vi "mini_test_app_serial_gpib.vi"() -> ()   [LabVIEW 2015]
doc: "Mini test app"
uses:
  Type Definitions/Highway_GB_Data.ctl
  Type Definitions/Highway_HP_Data.ctl
panel:
  out "HP ID":string="\r\n" caption="Hi-Pot Instrument ID"
  out "GB ID":string="\r\n" caption="GB Instrument ID"
  out "I/F type":string caption="Interface type"
  out "Results GB":string
  out "Status GB":string
  in  "Stop GB":bool
  in  "Start GB":bool
  in  "Stop Hi-Pot":bool
  out "Results HP":string
  in  "Exit Button":bool
  in  "Start Hi-Pot":bool
  out "Status HP":string
  # "Warning. This app is a proof of concept and has no other purpose, \nit is not intended for production. Likewise, it has no error handling. \nUse at your own risk."
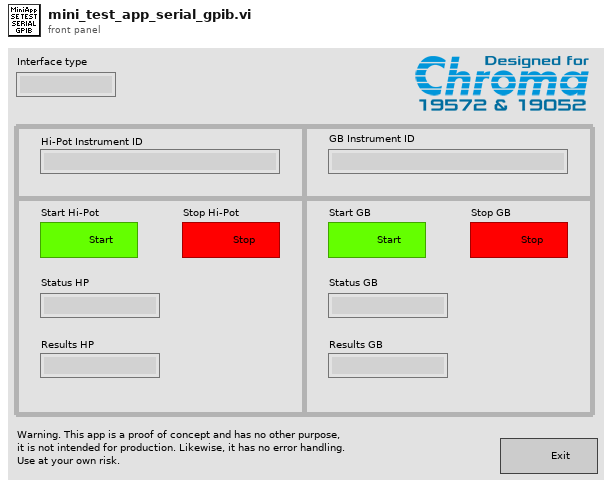
[diagram p1: front panel]
types:
  T1 = typedef "Highway_HP_Data.ctl" = cluster{"Status HP":string, "Results HP":string}
  T2 = typedef "Highway_GB_Data.ctl" = cluster{"Status GB":string, "Results GB":string}
  T3 = cluster{"VISA1 Inst ID":string, "VISA2 Inst ID":string, "I/F type":string}
  T4 = cluster{"Rsrc name for 19572":refnum<visa-resource-name>, "Rsrc name for 19052":refnum<visa-resource-name>}
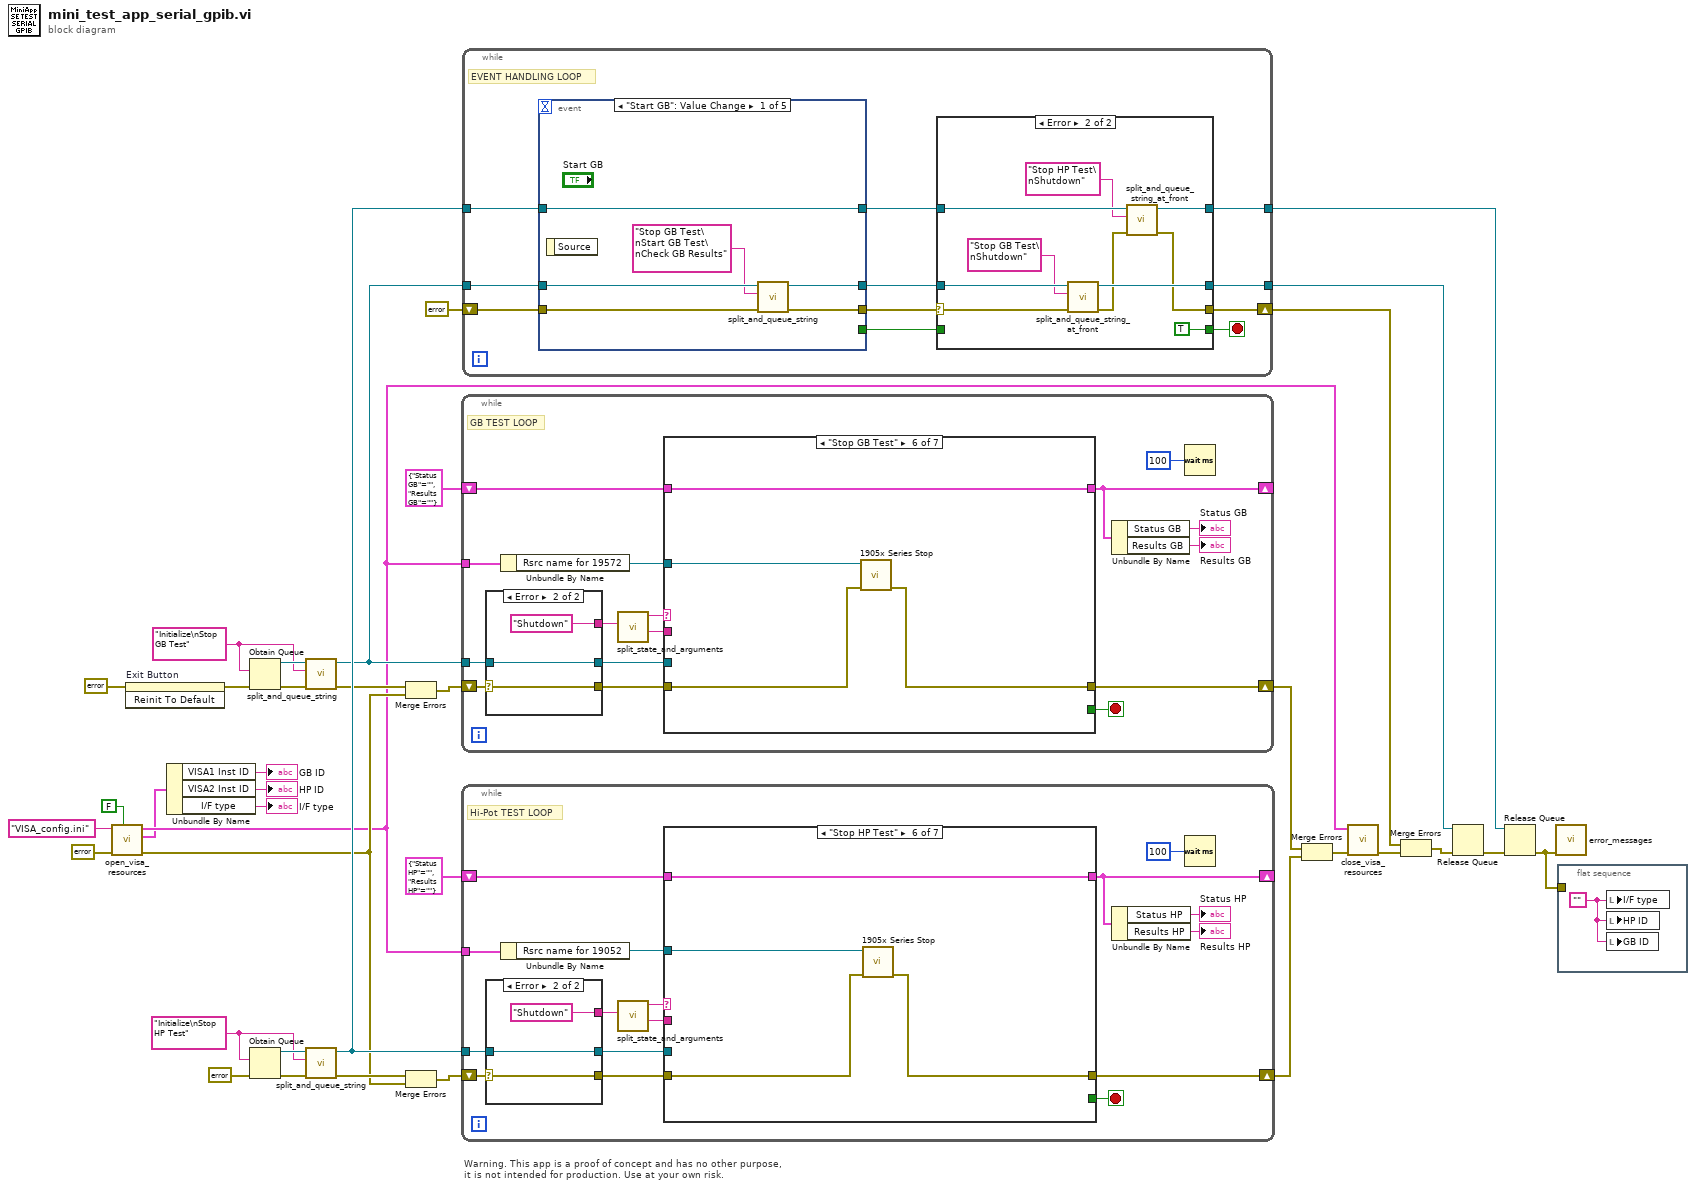
[diagram p0: block diagram]
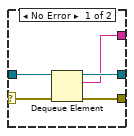
[diagram p2: hidden frame]
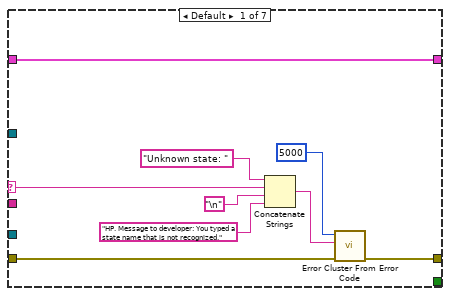
[diagram p3: hidden frame]
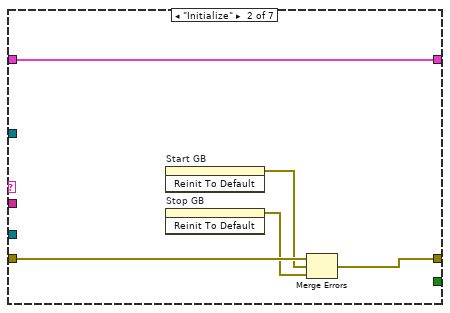
[diagram p4: hidden frame]
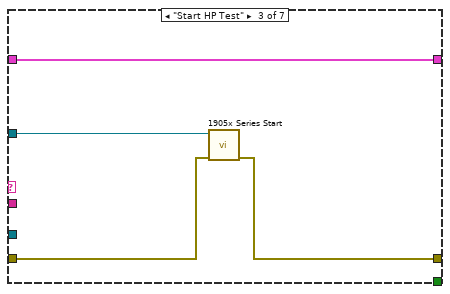
[diagram p5: hidden frame]
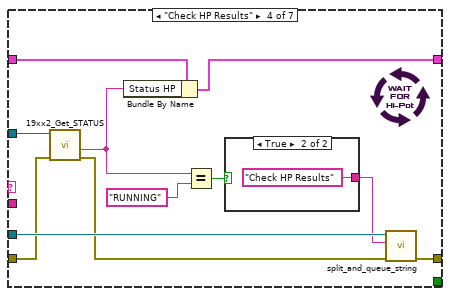
[diagram p6: hidden frame]
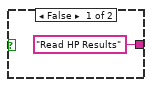
[diagram p7: hidden frame]
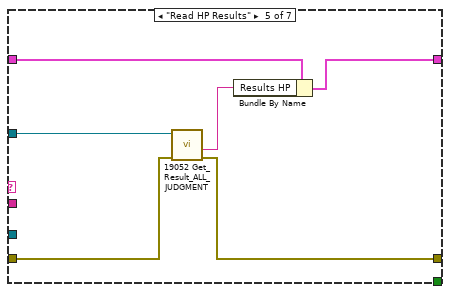
[diagram p8: hidden frame]
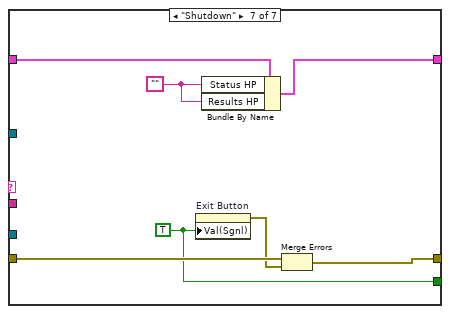
[diagram p9: hidden frame]
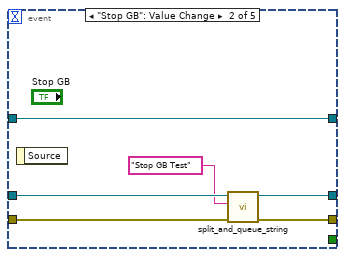
[diagram p11: hidden frame]
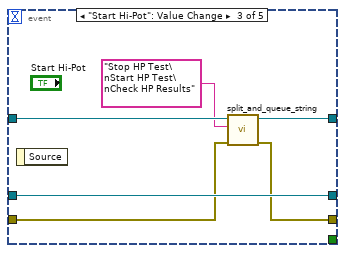
[diagram p12: hidden frame]
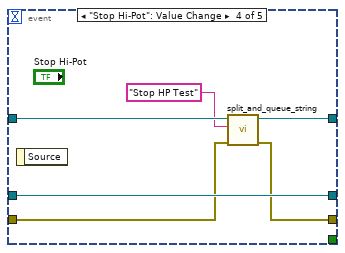
[diagram p13: hidden frame]
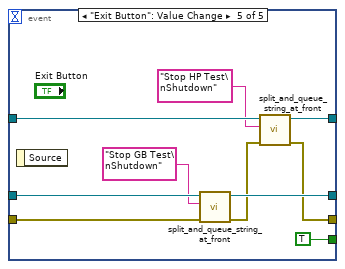
[diagram p14: hidden frame]
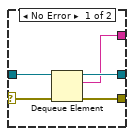
[diagram p15: hidden frame]
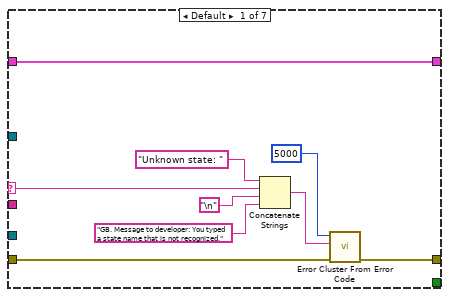
[diagram p16: hidden frame]
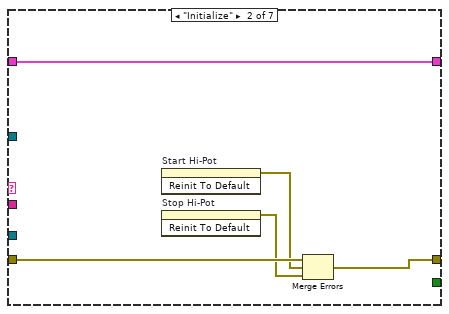
[diagram p17: hidden frame]
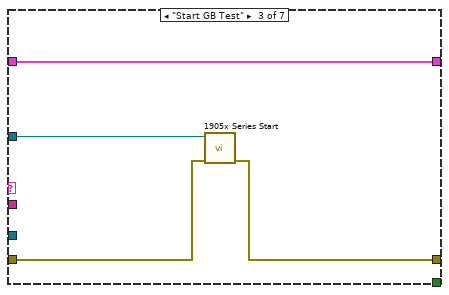
[diagram p18: hidden frame]
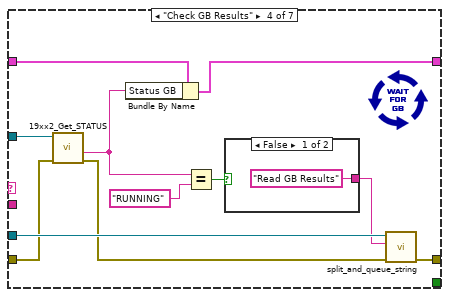
[diagram p19: hidden frame]
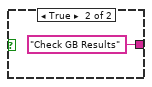
[diagram p20: hidden frame]
diagram:
  w13 = "Initialize\nStop HP Test" ("program string")
  w32 = "Initialize\nStop GB Test" ("program string")
  # "Warning. This app is a proof of concept and has no other purpose, \nit is not intended for production. Use at your own risk."
  n1 = call "open_visa_resources.vi"("test mode"=FALSE, "error in (no error)"=errorcluster {"status"=FALSE, "code"=0, "source"=""} ("error constant"), "config file in"="VISA_config.ini") -> ("error out"=w8:errorcluster, "Assgs"=w2:T3, "VISA"=w5:T4)  [unwired: 6 in]
  n2 = invoke on="Exit Button" class="Bool (strict)" method="Reinit To Default"(error in=errorcluster {"status"=FALSE, "code"=0, "source"=""} ("error constant")) -> (error out=w16:errorcluster)  [unwired: 2 in, 2 out]
  n3 = Unbundle By Name(w2) -> ("VISA1 Inst ID"=→"GB ID":string, "VISA2 Inst ID"=→"HP ID":string, "I/F type"=→"I/F type":string)
  n4 = Obtain Queue(element data type=w32, error in (no error)=w16) -> (queue out=w36:refnum<queue>, error out=w35:errorcluster)  [unwired: 3 in, 1 out]
  n5 = Obtain Queue(element data type=w13, error in (no error)=errorcluster {"status"=FALSE, "code"=0, "source"=""} ("error constant")) -> (queue out=w20:refnum<queue>, error out=w22:errorcluster)  [unwired: 3 in, 1 out]
  n6 = call "split_and_queue_string.vi"("error in (no error)"=w35, "program string"=w32, "queue in"=w36) -> ("error out"=w7:errorcluster, "queue out"=w31:refnum<queue>)  [unwired: 7 in]
  n7 = call "split_and_queue_string.vi"("error in (no error)"=w22, "program string"=w13, "queue in"=w20) -> ("error out"=w23:errorcluster, "queue out"=w37:refnum<queue>)  [unwired: 7 in]
  n8 = Merge Errors(w7, w8) -> (w28:errorcluster)
  n9 = Merge Errors(w23, w8) -> (w21:errorcluster)
  n10 = while {
    shift-right: [w51] -> w10
    shift-left: w28 -> [w44]
    tunnel: w31 -> [w45]
    tunnel: w5 -> [w39]
    shift-right: [w42] -> _
    shift-left: T2 {"Status GB"="", "Results GB"=""} -> [w43]
    stop <- w47 stop-if-true
    # "GB TEST LOOP"
    n11 = case shown="Error" w44 {
      selector: w44 -> [w58 w61]
      tunnel: [w57 w61] -> w52
      tunnel: w45 -> [w54 w60]
      tunnel: [w56 w60] -> w46
      tunnel: [w55 "Shutdown"] -> w49
      frame No Error {
        n12 = Dequeue Element(queue=w54, error in (no error)=w58) -> (queue out=w56:refnum<queue>, element=w55:string, error out=w57:errorcluster)  [unwired: 1 in, 1 out]
      }
      frame Error {
      }
    }
    n13 = Unbundle By Name(w39) -> ("Rsrc name for 19572"=w38:refnum<visa-resource-name>)
    n14 = call "split_state_and_arguments.vi"("String"=w49) -> ("Arguments"=w48:string, "State"=w50:string)  [unwired: 9 in]
    n15 = case shown="\"Stop GB Test\"" w50 {
      selector: w50 -> [w66 _ _ _ _ _ _]
      tunnel: [w64 w74 w79 w86 w97 w101 w107] -> w51
      tunnel: w52 -> [w65 w73 w78 w89 w98 w102 w109]
      tunnel: w46 -> [_ _ _ w90 _ _ _]
      tunnel: w48 -> [_ _ _ _ _ _ _]
      tunnel: [_ _ _ _ _ _ w108] -> w47
      tunnel: w38 -> [_ _ w77 w83 w96 w100 _]
      tunnel: w43 -> [w62 w75 w76 w82 w95 w99 w105]
      tunnel: [w62 w75 w76 w81 w94 w99 w104] -> w42
      frame Default {
        n16 = Concatenate Strings("Unknown state: " ("string"), w66, "\n", "GB. Message to developer: You typed a state name that is not recognized.") -> (w68:string)
        n17 = call <vilib>:"Error Cluster From Error Code.vi"("error in (no error)"=w65, "error message (\"\")"=w68, "error code (0)"=5000) -> ("error out"=w64:errorcluster)  [unwired: 6 in]
      }
      frame "Initialize" {
        n18 = invoke on="Start Hi-Pot" class="Bool" method="Reinit To Default"() -> (error out=w72:errorcluster)  [unwired: 3 in, 2 out]
        n19 = invoke on="Stop Hi-Pot" class="Bool" method="Reinit To Default"() -> (error out=w71:errorcluster)  [unwired: 3 in, 2 out]
        n20 = Merge Errors(w73, w72, w71) -> (w74:errorcluster)
      }
      frame "Start GB Test" {
        n21 = call "1905x Series Start.vi"("error in (no error)"=w78, "VISA resource in"=w77) -> ("error out"=w79:errorcluster)  [unwired: 8 in, 1 out]
      }
      frame "Check GB Results" {
        n22 = call "19xx2_Get_STATUS.vi"("error in (no error)"=w89, "VISA resource in"=w83) -> ("error out"=w87:errorcluster, "Status"=w80:string)  [unwired: 7 in, 1 out]
        n23 = Bundle By Name(cluster=w82, "Status GB"=w80) -> (w81:T2)
        n24 = Equal?(x=w80, y="RUNNING") -> (x = y?=w84:bool)
        n25 = case shown="False" w84 {
          tunnel: ["Read GB Results" ("program string") "Check GB Results" ("program string")] -> w85
          frame False {
          }
          frame True {
          }
        }
        n26 = call "split_and_queue_string.vi"("error in (no error)"=w87, "program string"=w85, "queue in"=w90) -> ("error out"=w86:errorcluster)  [unwired: 7 in, 1 out]
      }
      frame "Read GB Results" {
        n27 = call "19052 Get_Result_ALL_JUDGMENT.vi"("error in (no error)"=w98, "VISA resource in"=w96) -> ("error out"=w97:errorcluster, "JUDGMENT"=w93:string)  [unwired: 7 in, 1 out]
        n28 = Bundle By Name(cluster=w95, "Results GB"=w93) -> (w94:T2)
      }
      frame "Stop GB Test" {
        n29 = call "1905x Series Stop.vi"("error in (no error)"=w102, "VISA resource in"=w100) -> ("error out"=w101:errorcluster)  [unwired: 8 in, 1 out]
      }
      frame "Shutdown" {
        w103 = ""
        w108 = TRUE
        n30 = Bundle By Name(cluster=w105, "Status GB"=w103, "Results GB"=w103) -> (w104:T2)
        n31 = property on="Exit Button" class="Bool (strict)"("Val(Sgnl)"=w108) -> (error out=w106:errorcluster)  [unwired: 2 in, 1 out]
        n32 = Merge Errors(w109, w106) -> (w107:errorcluster)
      }
    }
    n33 = Unbundle By Name(w42) -> ("Status GB"=→"Status GB":string, "Results GB"=→"Results GB":string)
    n34 = Wait (ms)(milliseconds to wait=u32 100) -> ()  [unwired: 1 out]
  }
  n35 = while {
    shift-right: [w123] -> w3
    shift-left: w21 -> [w116]
    tunnel: w37 -> [w117]
    tunnel: w5 -> [w111]
    shift-right: [w114] -> _
    shift-left: T1 {"Status HP"="", "Results HP"=""} -> [w115]
    stop <- w119 stop-if-true
    # "Hi-Pot TEST LOOP"
    n36 = case shown="Error" w116 {
      selector: w116 -> [w130 w133]
      tunnel: [w129 w133] -> w124
      tunnel: w117 -> [w126 w132]
      tunnel: [w128 w132] -> w118
      tunnel: [w127 "Shutdown"] -> w121
      frame No Error {
        n37 = Dequeue Element(queue=w126, error in (no error)=w130) -> (queue out=w128:refnum<queue>, element=w127:string, error out=w129:errorcluster)  [unwired: 1 in, 1 out]
      }
      frame Error {
      }
    }
    n38 = Unbundle By Name(w111) -> ("Rsrc name for 19052"=w110:refnum<visa-resource-name>)
    n39 = call "split_state_and_arguments.vi"("String"=w121) -> ("Arguments"=w120:string, "State"=w122:string)  [unwired: 9 in]
    n40 = case shown="\"Stop HP Test\"" w122 {
      selector: w122 -> [w138 _ _ _ _ _ _]
      tunnel: [w136 w146 w151 w157 w168 w172 w179] -> w123
      tunnel: w124 -> [w137 w145 w149 w160 w169 w173 w181]
      tunnel: w118 -> [_ _ _ w162 _ _ _]
      tunnel: w120 -> [_ _ _ _ _ _ _]
      tunnel: w110 -> [_ _ w150 w161 w170 w174 _]
      tunnel: [_ _ _ _ _ _ w180] -> w119
      tunnel: w115 -> [w134 w147 w148 w154 w167 w171 w177]
      tunnel: [w134 w147 w148 w153 w166 w171 w176] -> w114
      frame Default {
        n41 = Concatenate Strings("Unknown state: " ("string"), w138, "\n", "HP. Message to developer: You typed a state name that is not recognized.") -> (w140:string)
        n42 = call <vilib>:"Error Cluster From Error Code.vi"("error in (no error)"=w137, "error message (\"\")"=w140, "error code (0)"=5000) -> ("error out"=w136:errorcluster)  [unwired: 6 in]
      }
      frame "Initialize" {
        n43 = invoke on="Start GB" class="Bool" method="Reinit To Default"() -> (error out=w144:errorcluster)  [unwired: 3 in, 2 out]
        n44 = invoke on="Stop GB" class="Bool" method="Reinit To Default"() -> (error out=w143:errorcluster)  [unwired: 3 in, 2 out]
        n45 = Merge Errors(w145, w144, w143) -> (w146:errorcluster)
      }
      frame "Start HP Test" {
        n46 = call "1905x Series Start.vi"("error in (no error)"=w149, "VISA resource in"=w150) -> ("error out"=w151:errorcluster)  [unwired: 8 in, 1 out]
      }
      frame "Check HP Results" {
        n47 = call "19xx2_Get_STATUS.vi"("error in (no error)"=w160, "VISA resource in"=w161) -> ("error out"=w158:errorcluster, "Status"=w152:string)  [unwired: 7 in, 1 out]
        n48 = Bundle By Name(cluster=w154, "Status HP"=w152) -> (w153:T1)
        n49 = Equal?(x=w152, y="RUNNING") -> (x = y?=w155:bool)
        n50 = case shown="True" w155 {
          tunnel: ["Read HP Results" ("program string") "Check HP Results" ("program string")] -> w156
          frame False {
          }
          frame True {
          }
        }
        n51 = call "split_and_queue_string.vi"("error in (no error)"=w158, "program string"=w156, "queue in"=w162) -> ("error out"=w157:errorcluster)  [unwired: 7 in, 1 out]
      }
      frame "Read HP Results" {
        n52 = call "19052 Get_Result_ALL_JUDGMENT.vi"("error in (no error)"=w169, "VISA resource in"=w170) -> ("error out"=w168:errorcluster, "JUDGMENT"=w165:string)  [unwired: 7 in, 1 out]
        n53 = Bundle By Name(cluster=w167, "Results HP"=w165) -> (w166:T1)
      }
      frame "Stop HP Test" {
        n54 = call "1905x Series Stop.vi"("error in (no error)"=w173, "VISA resource in"=w174) -> ("error out"=w172:errorcluster)  [unwired: 8 in, 1 out]
      }
      frame "Shutdown" {
        w175 = ""
        w180 = TRUE
        n55 = property on="Exit Button" class="Bool (strict)"("Val(Sgnl)"=w180) -> (error out=w178:errorcluster)  [unwired: 2 in, 1 out]
        n56 = Bundle By Name(cluster=w177, "Status HP"=w175, "Results HP"=w175) -> (w176:T1)
        n57 = Merge Errors(w181, w178) -> (w179:errorcluster)
      }
    }
    n58 = Unbundle By Name(w114) -> ("Status HP"=→"Status HP":string, "Results HP"=→"Results HP":string)
    n59 = Wait (ms)(milliseconds to wait=u32 100) -> ()  [unwired: 1 out]
  }
  n60 = while {
    tunnel: w31 -> [w191]
    tunnel: [w187] -> w33
    shift-right: [w190] -> w34
    shift-left: errorcluster {"status"=FALSE, "code"=0, "source"=""} ("error constant") -> [w192]
    tunnel: w37 -> [w184]
    tunnel: [w182] -> w14
    stop <- w188 stop-if-true
    # "EVENT HANDLING LOOP"
    n61 = event shown="[0] \"Start GB\": Value Change" {
      selector: _ -> [_ _ _ _ _]
      dyn-events: _ -> [_ _ _ _ _]
      timeout: _ -> [_ _ _ _ _]
      tunnel: w191 -> [w210 w215 w224 w230 w238]
      tunnel: w192 -> [w209 w217 w223 w229 w235]
      tunnel: [w211 w218 w222 w228 w231] -> w185
      tunnel: [_ _ _ _ TRUE] -> w189
      tunnel: [w212 w216 w224 w230 w239] -> w186
      tunnel: w184 -> [w207 w213 w221 w227 w237]
      tunnel: [w207 w213 w219 w225 w236] -> w183
      event "Start GB": Value Change {
        n62 = event-data() -> ()  [unwired: 1 in, 1 out]
        n63 = call "split_and_queue_string.vi"("error in (no error)"=w209, "program string"="Stop GB Test\nStart GB Test\nCheck GB Results", "queue in"=w210) -> ("error out"=w211:errorcluster, "queue out"=w212:refnum<queue>)  [unwired: 7 in]
      }
      event "Stop GB": Value Change {
        n64 = event-data() -> ()  [unwired: 1 in, 1 out]
        n65 = call "split_and_queue_string.vi"("error in (no error)"=w217, "program string"="Stop GB Test", "queue in"=w215) -> ("error out"=w218:errorcluster, "queue out"=w216:refnum<queue>)  [unwired: 7 in]
      }
      event "Start Hi-Pot": Value Change {
        n66 = event-data() -> ()  [unwired: 1 in, 1 out]
        n67 = call "split_and_queue_string.vi"("error in (no error)"=w223, "program string"="Stop HP Test\nStart HP Test\nCheck HP Results", "queue in"=w221) -> ("error out"=w222:errorcluster, "queue out"=w219:refnum<queue>)  [unwired: 7 in]
      }
      event "Stop Hi-Pot": Value Change {
        n68 = event-data() -> ()  [unwired: 1 in, 1 out]
        n69 = call "split_and_queue_string.vi"("error in (no error)"=w229, "program string"="Stop HP Test", "queue in"=w227) -> ("error out"=w228:errorcluster, "queue out"=w225:refnum<queue>)  [unwired: 7 in]
      }
      event "Exit Button": Value Change {
        n70 = event-data() -> ()  [unwired: 1 in, 1 out]
        n71 = call "split_and_queue_string_at_front.vi"("error in (no error)"=w235, "program string"="Stop GB Test\nShutdown", "queue in"=w238) -> ("error out"=w233:errorcluster, "queue out"=w239:refnum<queue>)  [unwired: 7 in]
        n72 = call "split_and_queue_string_at_front.vi"("error in (no error)"=w233, "program string"="Stop HP Test\nShutdown", "queue in"=w237) -> ("error out"=w231:errorcluster, "queue out"=w236:refnum<queue>)  [unwired: 7 in]
      }
    }
    n73 = case shown="Error" w185 {
      selector: w185 -> [w196 w205]
      tunnel: [w196 w198] -> w190
      tunnel: w189 -> [w195 _]
      tunnel: [w195 TRUE] -> w188
      tunnel: [w194 w204] -> w187
      tunnel: w186 -> [w194 w203]
      tunnel: w183 -> [w193 w201]
      tunnel: [w193 w200] -> w182
      frame No Error {
      }
      frame Error {
        n74 = call "split_and_queue_string_at_front.vi"("error in (no error)"=w205, "program string"="Stop GB Test\nShutdown", "queue in"=w203) -> ("error out"=w199:errorcluster, "queue out"=w204:refnum<queue>)  [unwired: 7 in]
        n75 = call "split_and_queue_string_at_front.vi"("error in (no error)"=w199, "program string"="Stop HP Test\nShutdown", "queue in"=w201) -> ("error out"=w198:errorcluster, "queue out"=w200:refnum<queue>)  [unwired: 7 in]
      }
    }
  }
  n76 = Merge Errors(w10, w3) -> (w4:errorcluster)
  n77 = call "close_visa_resources.vi"("error in (no error)"=w4, "VISA"=w5) -> ("error out"=w12:errorcluster)  [unwired: 9 in]
  n78 = Merge Errors(w34, w12) -> (w9:errorcluster)
  n79 = Release Queue(queue=w33, error in (no error)=w9) -> (error out=w15:errorcluster)  [unwired: 1 in, 2 out]
  n80 = Release Queue(queue=w14, error in (no error)=w15) -> (error out=w1:errorcluster)  [unwired: 1 in, 2 out]
  n81 = call "error_messages.vi"("error in (no error)"=w1) -> ()  [unwired: 11 in]
  n82 = flat-sequence {
    tunnel: w1 -> [_]
    frame #0 {
      w241 = ""
      n83 = local write "I/F type"(w241) -> ()
      n84 = local write "HP ID"(w241) -> ()
      n85 = local write "GB ID"(w241) -> ()
    }
  }
